vi "PAN_DBS_is_queued.vi"(10 "args in":string) -> (1 "queue?":bool, 2 "args out":string)   [LabVIEW 2016]
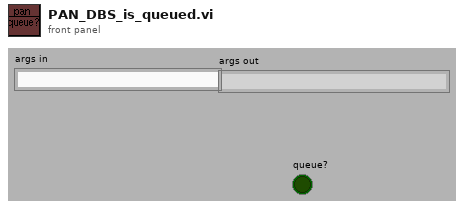
[diagram p1: front panel]
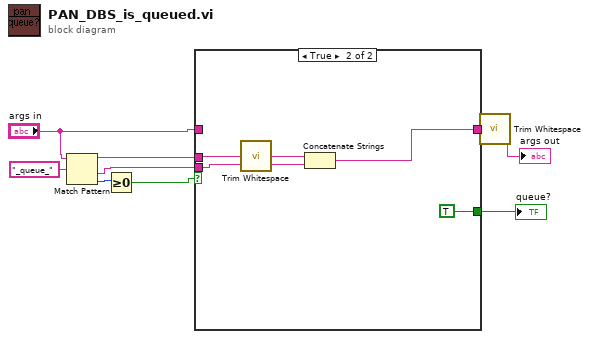
[diagram p0: block diagram]
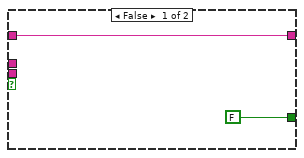
[diagram p2: hidden frame]
diagram:
  n1 = Match Pattern(string="args in", regular expression="_queue_") -> (before substring=w5:string, after substring=w4:string, offset past match=w8:i32)  [unwired: 2 out]
  n2 = Greater Or Equal To 0?(x=w8) -> (x >= 0?=w1:bool)
  n3 = case shown="True" w1 {
    tunnel: "args in" -> [w11 _]
    tunnel: [w11 w14] -> w7
    tunnel: [FALSE ("queue?") TRUE ("queue?")] -> w6
    tunnel: w5 -> [_ w16]
    tunnel: w4 -> [_ w15]
    frame False {
    }
    frame True {
      n4 = call <vilib>:"Trim Whitespace.vi"("string"=w16) -> ("trimmed string"=w12:string)  [unwired: 1 in]
      n5 = Concatenate Strings(w12, w15) -> (w14:string)
    }
  }
  "queue?" <- w6
  n6 = call <vilib>:"Trim Whitespace.vi"("string"=w7) -> ("trimmed string"=→"args out":string)  [unwired: 1 in]
